vi "Global micro_Devices.vi"() -> ()   [LabVIEW 2021]
panel:
  out "microfabricating":bool
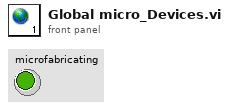
[diagram p1: front panel]
diagram:
